vi "AuMT8852B CW Measurement Results Query.vi"(8 "error in (no error)":errorcluster, 11 "VISA session":refnum<visa-resource-name>) -> (0 "error out":errorcluster, 2 "error code":i32, 3 "VISA session out":refnum<visa-resource-name>, 4 "Results":T1 {"Max negative deviation (kHz)" format="%.2f"; "Max positive deviation (kHz)" format="%.2f"; "Power (dBm)" format="%.2f"; "Frequency offset (kHz)" format="%.2f"})   [LabVIEW 2017]
doc: "Anritsu MT8852B Bluetooth Tester\n\nReturns the results of the CW measurement.\n\nOUTPUTS\nResults - measurements made during the test."
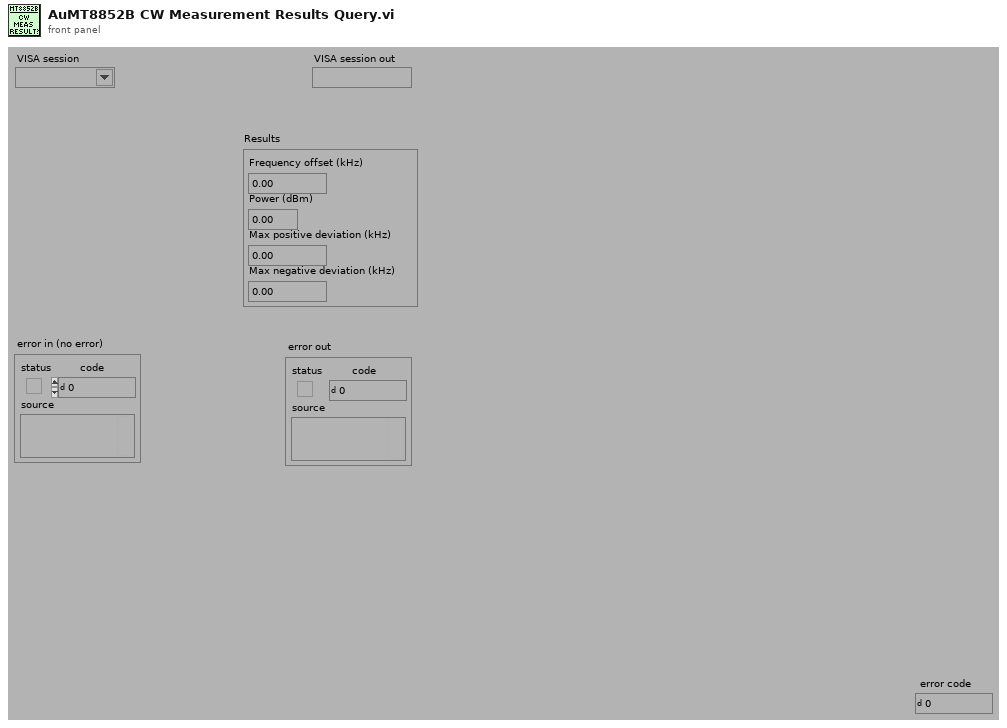
[diagram p1: front panel]
types:
  T1 = cluster{"Frequency offset (kHz)":dbl, "Power (dBm)":dbl, "Max positive deviation (kHz)":dbl, "Max negative deviation (kHz)":dbl}
  T2 = enum16{"Simulate", "Range check", "Cache", "Query instrument status"}
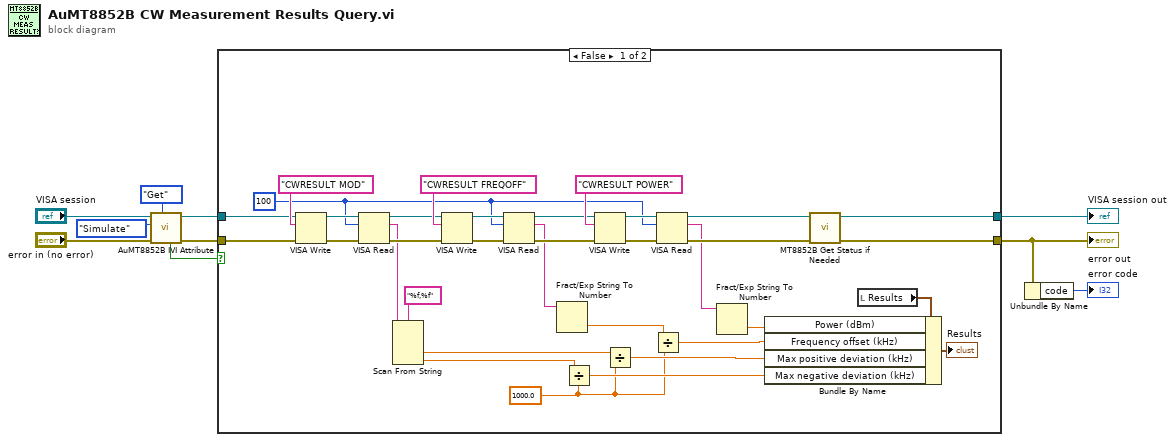
[diagram p0: block diagram]
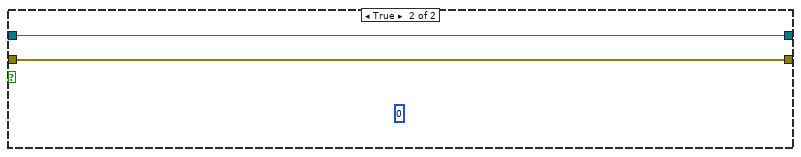
[diagram p2: hidden frame]
diagram:
  n1 = call <instrlib>:"AuMT8852B IVI Attribute.vi"("Set/Get (Set)"=enum16{"Set", "Get"}."Get", "error in (no error)"="error in (no error)", "Flag (Simulate)"=T2."Simulate", "VISA session"="VISA session") -> ("error out"=w7:errorcluster, "VISA session out"=w9:refnum<visa-resource-name>, "Value out"=w3:bool)  [unwired: 5 in]
  n2 = case shown="False" w3 {
    tunnel: [w37 w46] -> w10
    tunnel: [w36 w45] -> w1
    tunnel: w9 -> [w43 w46]
    tunnel: w7 -> [w42 w45]
    frame False {
      w13 = 1000.0 ("y")
      w11 = u32 100 ("byte count (0)")
      n3 = VISA Write(VISA resource name=w43, write buffer="CWRESULT MOD" ("write buffer (\"\")"), error in (no error)=w42) -> (VISA resource name out=w41:refnum<visa-resource-name>, error out=w40:errorcluster)  [unwired: 1 out]
      n4 = VISA Read(VISA resource name=w41, byte count=w11, error in (no error)=w40) -> (VISA resource name out=w33:refnum<visa-resource-name>, read buffer=w22:string, error out=w32:errorcluster)  [unwired: 1 out]
      n5 = Scan From String(format string="%f,%f" ("Format String"), input string=w22) -> (output 1=w19:dbl, output 2=w21:dbl)  [unwired: 4 in, 3 out]
      n6 = VISA Write(VISA resource name=w33, write buffer="CWRESULT FREQOFF" ("write buffer (\"\")"), error in (no error)=w32) -> (VISA resource name out=w35:refnum<visa-resource-name>, error out=w31:errorcluster)  [unwired: 1 out]
      n7 = VISA Read(VISA resource name=w35, byte count=w11, error in (no error)=w31) -> (VISA resource name out=w26:refnum<visa-resource-name>, read buffer=w17:string, error out=w27:errorcluster)  [unwired: 1 out]
      n8 = Fract/Exp String To Number(string=w17) -> (number=w16:dbl)  [unwired: 3 in, 1 out]
      n9 = Divide(x=w21, y=w13) -> (x/y=w20:dbl)
      n10 = VISA Write(VISA resource name=w26, write buffer="CWRESULT POWER" ("write buffer (\"\")"), error in (no error)=w27) -> (VISA resource name out=w28:refnum<visa-resource-name>, error out=w30:errorcluster)  [unwired: 1 out]
      n11 = Divide(x=w19, y=w13) -> (x/y=w18:dbl)
      n12 = Divide(x=w16, y=w13) -> (x/y=w14:dbl)
      n13 = VISA Read(VISA resource name=w28, byte count=w11, error in (no error)=w30) -> (VISA resource name out=w23:refnum<visa-resource-name>, read buffer=w15:string, error out=w24:errorcluster)  [unwired: 1 out]
      n14 = Fract/Exp String To Number(string=w15) -> (number=w12:dbl)  [unwired: 3 in, 1 out]
      n15 = call <instrlib>:"MT8852B Get Status if Needed.vi"("error in (no error)"=w24, "VISA session"=w23) -> ("error out"=w36:errorcluster, "VISA session out"=w37:refnum<visa-resource-name>)  [unwired: 8 in]
      n16 = local read "Results"() -> (w39:T1)
      n17 = Bundle By Name(cluster=w39, "Power (dBm)"=w12, "Frequency offset (kHz)"=w14, "Max positive deviation (kHz)"=w18, "Max negative deviation (kHz)"=w20) -> (→"Results":T1)
    }
    frame True {
      (unwired) u8 0
    }
  }
  "error out" <- w1
  "VISA session out" <- w10
  n18 = Unbundle By Name(w1) -> ("code"=→"error code":i32)
